vi "BRig_RT__Case_Exp__State_RewardPre.vi"(0 "input_dataCurrent":u16[](array[numeric]), 9 "input_dataBlock":u16[][](array[numeric]), 11 "input_dataTrial":u16[][](array[numeric])) -> (1 "output_T_Reward":u16, 2 "output_c_nReward_total_R":u16, 3 "output_c_nReward_total_L":u16, 4 "output_dataCurrent":u16[](array[numeric]), 10 "output_dataBlock":u16[][](array[numeric]), 13 "output_c_nReward_total":u16, 14 "output_nReward":u16, 15 "output_dataTrial":u16[][](array[numeric]))   [LabVIEW 2014]
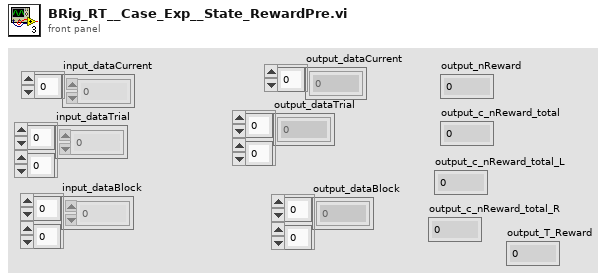
[diagram p1: front panel]
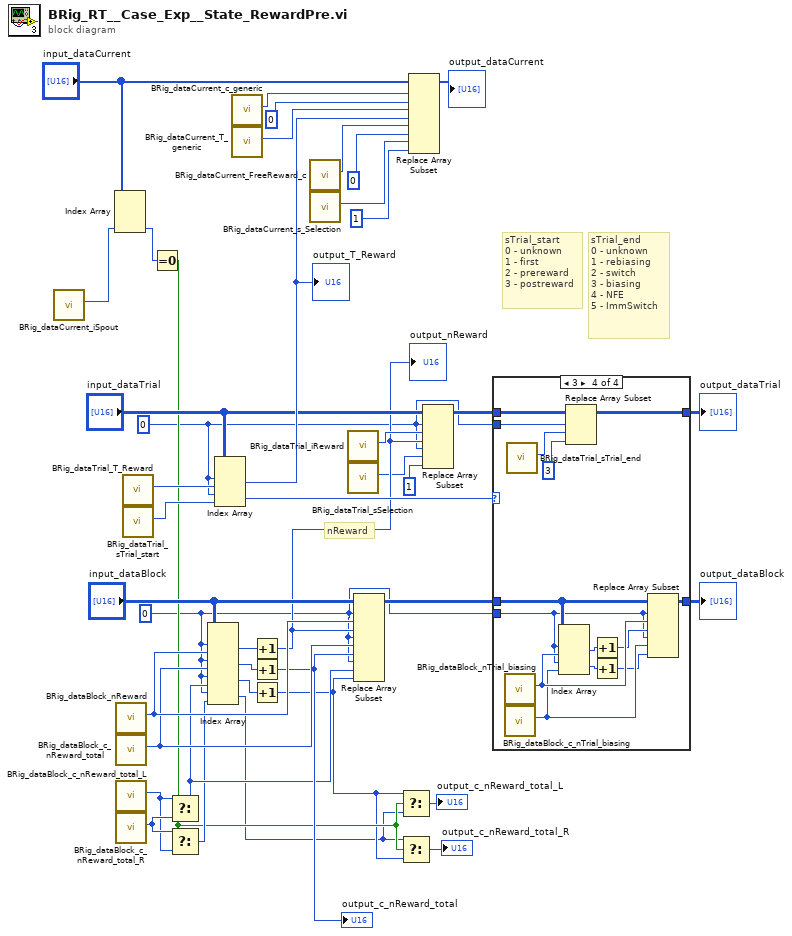
[diagram p0: block diagram]
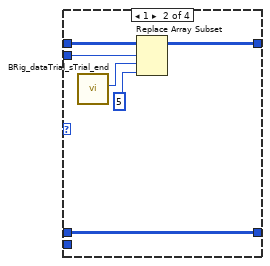
[diagram p3: hidden frame]
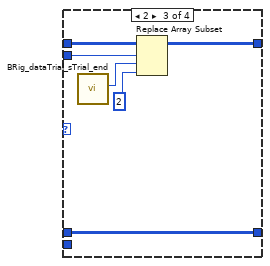
[diagram p4: hidden frame]
diagram:
  w2 = 0
  w1 = 0
  # "nReward"
  # "sTrial_end\n0 - unknown\n1 - rebiasing\n2 - switch\n3 - biasing\n4 - NFE\n5 - ImmSwitch"
  # "sTrial_start\n0 - unknown\n1 - first\n2 - prereward\n3 - postreward"
  n1 = call "BRig_dataCurrent_iSpout.vi"() -> ("output_iSpout"=w29:i32)  [unwired: 11 in]
  n2 = Index Array(array="input_dataCurrent", index #3=w29) -> (element #3=w28:u16)  [unwired: 2 in, 2 out]
  n3 = call "BRig_dataBlock_nReward.vi"() -> ("output_nReward"=w34:i32)  [unwired: 11 in]
  n4 = call "BRig_dataBlock_c_nReward_total.vi"() -> ("output_nReward_total"=w31:i32)  [unwired: 11 in]
  n5 = call "BRig_dataBlock_c_nReward_total_L.vi"() -> ("output_nReward_total_L"=w13:i32)  [unwired: 11 in]
  n6 = call "BRig_dataBlock_c_nReward_total_R.vi"() -> ("output_nReward_total_R"=w14:i32)  [unwired: 11 in]
  n7 = call "BRig_dataTrial_T_Reward.vi"() -> ("output_T_Reward"=w37:i32)  [unwired: 11 in]
  n8 = call "BRig_dataTrial_sTrial_start.vi"() -> ("output_sTrial_start"=w25:i32)  [unwired: 11 in]
  n9 = Equal To 0?(x=w28) -> (x = 0?=w11:bool)
  n10 = Select(t=w13, s=w11, f=w14) -> (s? t:f=w26:i32)
  n11 = Select(t=w14, s=w11, f=w13) -> (s? t:f=w12:i32)
  n12 = Index Array(array="input_dataBlock", index (row) #1=w1, index (col) #1=w34, index (row) #2=w1, index (col) #2=w31, index (row) #3=w1, index (col) #3=w26, index (row) #4=w1, index (col) #4=w12) -> (element #1=w33:u16, element #2=w32:u16, element #3=w27:u16, element #4=w9:u16)
  n13 = Index Array(array="input_dataTrial", index (row) #1=w2, index (col) #1=w37, index (row) #2=w2, index (col) #2=w25) -> (element #1=w36:u16, element #2=w24:u16)
  "output_T_Reward" <- w36
  n14 = call "BRig_dataCurrent_c_generic.vi"() -> ("output_count_generic"=w41:i32)  [unwired: 11 in]
  n15 = call "BRig_dataCurrent_T_generic.vi"() -> ("output_T_generic"=w40:i32)  [unwired: 11 in]
  n16 = Increment(x=w33) -> (x+1=w20:u16)
  "output_nReward" <- w20
  n17 = Increment(x=w32) -> (x+1=w30:u16)
  "output_c_nReward_total" <- w30
  n18 = Increment(x=w27) -> (x+1=w10:u16)
  n19 = call "BRig_dataCurrent_FreeReward_c.vi"() -> ("output_FreeReward_c"=w6:i32)  [unwired: 11 in]
  n20 = call "BRig_dataCurrent_s_Selection.vi"() -> ("output_s_Selection"=w4:i32)  [unwired: 11 in]
  n21 = call "BRig_dataTrial_iReward.vi"() -> ("output_iReward"=w21:i32)  [unwired: 11 in]
  n22 = call "BRig_dataTrial_sSelection.vi"() -> ("output_sSelection"=w16:i32)  [unwired: 11 in]
  n23 = Replace Array Subset(array="input_dataBlock", new element #1=w20, index (row) #1=w1, index (col) #1=w34, new element #2=w30, index (row) #2=w1, index (col) #2=w31, new element #3=w10, index (row) #3=w1, index (col) #3=w26) -> (w19:u16[][])
  n24 = Select(t=w10, s=w11, f=w9) -> (s? t:f=→"output_c_nReward_total_L":u16)
  n25 = Select(t=w9, s=w11, f=w10) -> (s? t:f=→"output_c_nReward_total_R":u16)
  n26 = Replace Array Subset(array="input_dataCurrent", new element #1=u16 0 ("new element/subarray"), index #1=w41, new element #2=w36, index #2=w40, new element #3=u16 0 ("new element/subarray"), index #3=w6, new element #4=u16 1 ("new element/subarray"), index #4=w4) -> (→"output_dataCurrent":u16[])
  n27 = Replace Array Subset(array="input_dataTrial", new element #1=w20, index (row) #1=w2, index (col) #1=w21, new element #2=u16 1 ("new element/subarray"), index (row) #2=w2, index (col) #2=w16) -> (w22:u16[][])
  n28 = case shown="3" w24 {
    tunnel: w22 -> [w44 w50 w56 w70]
    tunnel: w2 -> [_ w48 w54 w68]
    tunnel: [w44 w49 w55 w69] -> w17
    tunnel: w19 -> [w43 w45 w51 w64]
    tunnel: [w43 w45 w51 w65] -> w18
    tunnel: w1 -> [_ _ _ w60]
    frame 0, Default {
    }
    frame 1 {
      n29 = call "BRig_dataTrial_sTrial_end.vi"() -> ("output_sTrial_end"=w47:i32)  [unwired: 11 in]
      n30 = Replace Array Subset(array=w50, new element=u16 5 ("new element/subarray"), index (row)=w48, index (col)=w47) -> (w49:u16[][])
    }
    frame 2 {
      n31 = call "BRig_dataTrial_sTrial_end.vi"() -> ("output_sTrial_end"=w53:i32)  [unwired: 11 in]
      n32 = Replace Array Subset(array=w56, new element=u16 2 ("new element/subarray"), index (row)=w54, index (col)=w53) -> (w55:u16[][])
    }
    frame 3 {
      n33 = call "BRig_dataBlock_nTrial_biasing.vi"() -> ("output_nTrial_biasing"=w63:i32)  [unwired: 11 in]
      n34 = call "BRig_dataBlock_c_nTrial_biasing.vi"() -> ("output_c_nTrial_biasing"=w58:i32)  [unwired: 11 in]
      n35 = call "BRig_dataTrial_sTrial_end.vi"() -> ("output_sTrial_end"=w67:i32)  [unwired: 11 in]
      n36 = Index Array(array=w64, index (row) #1=w60, index (col) #1=w63, index (row) #2=w60, index (col) #2=w58) -> (element #1=w62:u16, element #2=w59:u16)
      n37 = Replace Array Subset(array=w70, new element=u16 3 ("new element/subarray"), index (row)=w68, index (col)=w67) -> (w69:u16[][])
      n38 = Increment(x=w62) -> (x+1=w61:u16)
      n39 = Increment(x=w59) -> (x+1=w57:u16)
      n40 = Replace Array Subset(array=w64, new element #1=w61, index (row) #1=w60, index (col) #1=w63, new element #2=w57, index (row) #2=w60, index (col) #2=w58) -> (w65:u16[][])
    }
  }
  "output_dataBlock" <- w18
  "output_dataTrial" <- w17
